vi "Get RD Data.vi"(8 "error in":errorcluster, 11 "tCRD in":refnum<class "Aircraft OPCCRD.lvclass">) -> (0 "error out":errorcluster, 3 "tCRD out":refnum<class "Aircraft OPCCRD.lvclass">)   [LabVIEW 2015, in "Aircraft OPCCRD.lvclass"]
uses:
  Aircraft OPCCRD.lvclass
  Aircraft OPCCRD.lvclass/Aircraft OPCCRD.ctl
  Reusable/Instrument/Instrument.lvclass/Instrument.ctl
  Reusable/CRDS/Main/CRDS.lvclass/CRDS.ctl
  Accessors/Read FPGA Ref.vi
  Accessors/Read RepRate.vi
  Accessors/Read SamplesPerRep.vi
  Reusable/Instrument/Write Restart Requested_.vi
  Reusable/CRDS/Main/Write Laser Data.vi
  <vilib>/Utility/error.llb/Error Cluster From Error Code.vi
  <vilib>/rvi/errors/niLvFpgaAdjustHostInterfaceError.vi
  tFPGA Ref.ctl
  <vilib>/rvi/interface/nirviMethod/nirviMethod.xnode
  FPGA Bitfiles/Aircraft OPCRD Server.lvbitx
  <vilib>/FPGAPlugInAG/sbRIO-9636/niLvFpga_ReadFifo_sbRIO-9636.vi
  <vilib>/rvi/errors/niLvFpgaMergeErrorWithErrorCode.vi
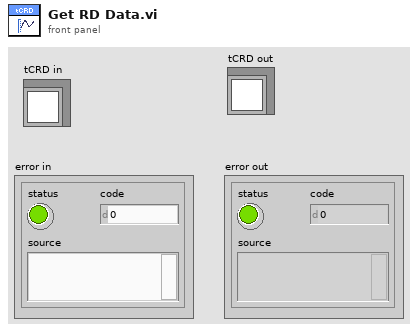
[diagram p1: front panel]
types:
  T1 = typedef "Aircraft OPCCRD.lvclass/tFPGA Ref.ctl" = refnum<k20>
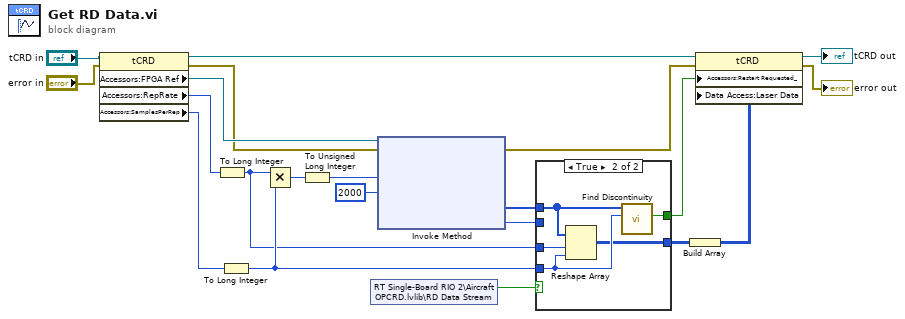
[diagram p0: block diagram]
diagram:
  n1 = property class="tCRD"(reference="tCRD in", error in="error in") -> (reference out=w1:refnum<class "Aircraft OPCCRD.lvclass">, error out=w4:errorcluster, "Accessors:FPGA Ref"=w12:T1, "Accessors:RepRate"=w14:u16, "Accessors:SamplesPerRep"=w13:u16)
  n2 = To Long Integer(number=w14) -> (32bit integer=w17:i32)
  n3 = To Long Integer(number=w13) -> (32bit integer=w21:i32)
  n4 = Multiply(x=w17, y=w21) -> (x*y=w16:i32)
  n5 = To Unsigned Long Integer(number=w16) -> (unsigned 32bit integer=w18:u32)
  n6 = shared-variable "RT Single-Board RIO 2\\Aircraft OPCRD.lvlib\\RD Data Stream"() -> (w6:bool)  [unwired: 1 in, 1 out]
  n7 = xnode "Invoke Method"("FPGA VI Reference In"=w12, "error in"=w4, "Number of Elements"=w18, "Timeout (ms)"=2000) -> ("error out"=w7:errorcluster, "Data"=w20:i16[], "Elements Remaining"=w2:u32)  [unwired: 1 out]
  n8 = case shown="True" w6 {
    tunnel: w17 -> [_ w26]
    tunnel: [_ w25] -> w11
    tunnel: w20 -> [_ w24]
    tunnel: w21 -> [_ w23]
    tunnel: [_ w22] -> w3
    tunnel: w2 -> [_ _]
    frame False {
    }
    frame True {
      n9 = Reshape Array(w24, w26, w23) -> (w22:i16[][])
      n10 = call "Find Discontinuity.vi"("Single Record"=w23, "Data"=w24) -> ("Discontinuity Detected"=w25:bool)  [unwired: 8 in, 1 out]
    }
  }
  n11 = Build Array(w3) -> (w10:i16[][][])
  n12 = property class="tCRD"(reference=w1, error in=w7, "Accessors:Restart Requested_"=w11, "Data Access:Laser Data"=w10) -> (reference out=→"tCRD out":refnum<class "Aircraft OPCCRD.lvclass">, error out=→"error out":errorcluster)
